vi "configure.vi"(8 "error in (no error)":errorcluster) -> (0 "error out":errorcluster, 1 "Track Division in Samples":i32, 2 "Track (File) References":T2, 3 "Refnum out":T1)   [LabVIEW 2014]
uses:
  Controls/Track (File) References.ctl
  Controls/FPGA Reference.ctl
  <vilib>/FPGAPlugInAG/myRIO-1900/niLvFpga_Open_myRIO-1900.vi
  <vilib>/rvi/interface/common/dynamic/niFpgaDynamicAddResources.vi
  <vilib>/rvi/interface/nirviOpenFPGA/nirviOpenFPGA.xnode
  FPGA Bitfiles/mySynth_FPGATarget_FPGAMain_huUPcriYQyU.lvbitx
  FPGA Main.vi
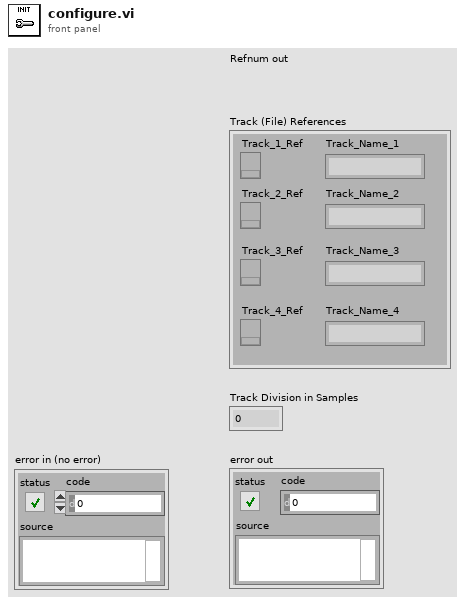
[diagram p1: front panel]
types:
  T1 = typedef "FPGA Reference.ctl" = refnum<k20>
  T2 = typedef "Track (File) References.ctl" = cluster{"Track_1_Ref":refnum<k34>, "Track_2_Ref":refnum<k34>, "Track_3_Ref":refnum<k34>, "Track_4_Ref":refnum<k34>, "Track_Name_1":string, "Track_Name_2":string, "Track_Name_3":string, "Track_Name_4":string}
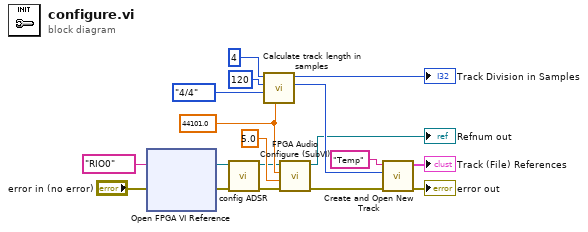
[diagram p0: block diagram]
diagram:
  w13 = 44101.0 ("Sample Rate (Hz)")
  n1 = xnode "Open FPGA VI Reference"("error in"="error in (no error)", "resource name"=tag "RIO0") -> ("FPGA VI Reference Out"=w5:refnum<k20>, "error out"=w4:errorcluster)
  n2 = call "config ADSR.vi"("error in (no error)"=w4, "Refnum in"=w5) -> ("error out"=w3:errorcluster, "Refnum out"=w2:refnum<k20>)  [unwired: 8 in]
  n3 = call "Calculate track length in samples.vi"("Sample Rate (Hz)"=w13, "Time Signature"=enum16{"4/4", "3/4"}."4/4", "BPM"=120, "Measures"=4) -> ("Track Length in Samples"=w17:i32, "Track Division in Samples"=→"Track Division in Samples":i32)  [unwired: 4 in, 2 out]
  n4 = call "FPGA Audio Configure (SubVI).vi"("error in (no error)"=w3, "Read Rate (Hz)"=5.0, "Audio Sample Rate (Hz)"=w13, "Refnum in"=w2) -> ("error out"=w11:errorcluster, "Refnum Out"=→"Refnum out":refnum<k20>)  [unwired: 4 in, 2 out]
  n5 = call "Create and Open New Track.vi"("Error In"=w11, "Samples Per Channel"=w17, "Track Name"="Temp") -> ("Error Out"=→"error out":errorcluster, "Track (File) References"=→"Track (File) References":T2)  [unwired: 7 in]
